vi "apply channel changes.vi"(8 "error in":errorcluster, 9 "new channel":refnum<class "TBM channel.lvclass">, 10 "old channel":refnum<class "TBM channel.lvclass">, 11 "alarms module configuration in":refnum<class "alarms module configuration.lvclass">=refnum) -> (0 "error out":errorcluster, 3 "alarms module configuration out":refnum<class "alarms module configuration.lvclass">)   [LabVIEW 2013]
doc: "Copyright 2016 National Instruments Corporation\n\nLicensed under the Apache License, Version 2.0 (the \"License\"); you may not use this file except in compliance with the License. You may obtain a copy of the License at http://www.apache.org/licenses/LICENSE-2.0\nUnless required by applicable law or agreed to in writing, software distributed under the License is distributed on an \"AS IS\" BASIS, WITHOUT WARRANTIES OR CONDITIONS OF ANY KIND, either express or implied. See the License for the specific language governing permissions and limitations under the License."
uses:
  <vilib>/NI/Tag Bus/tag/tag descriptor.lvclass
  alarms module configuration.lvclass
  <vilib>/NI/Tag Bus Module Framework/channel/TBM channel.lvclass
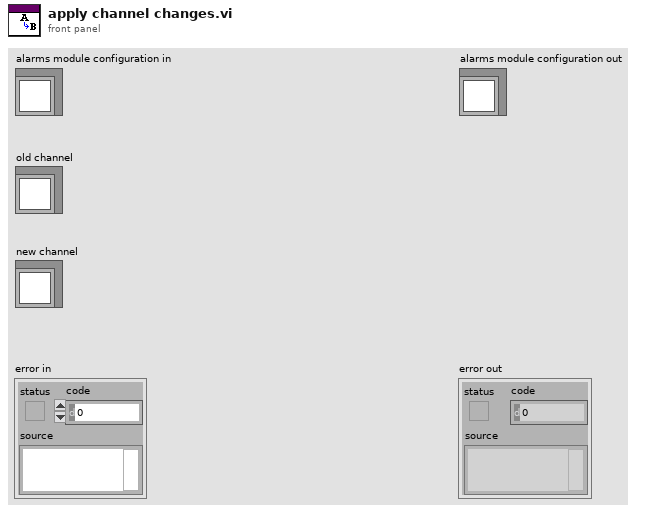
[diagram p1: front panel]
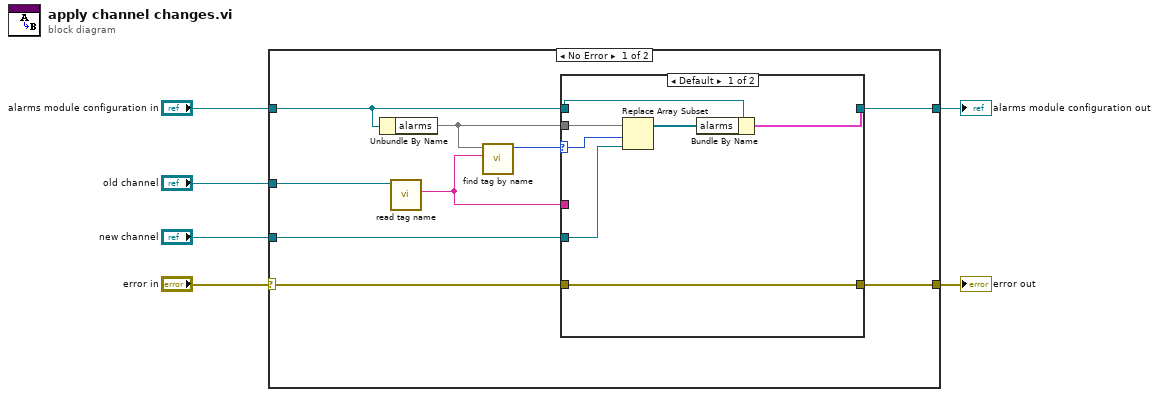
[diagram p0: block diagram]
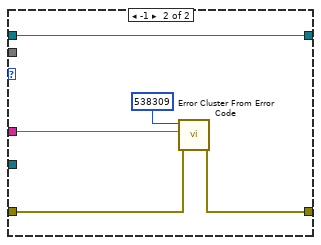
[diagram p2: hidden frame]
diagram:
  n1 = case shown="No Error" "error in" {
    selector: "error in" -> [w10 w29]
    tunnel: [w9 w29] -> w5
    tunnel: [w13 w28] -> w3
    tunnel: "alarms module configuration in" -> [w14 w28]
    tunnel: "old channel" -> [w15 _]
    tunnel: "new channel" -> [w11 _]
    frame No Error {
      n2 = Unbundle By Name(w14) -> ("alarms"=w12)
      n3 = call <vilib>:"read tag name.vi"("system tag in"=w15) -> ("name"=w7:string)  [unwired: 8 in, 2 out]
      n4 = call <vilib>:"find tag by name.vi"("name"=w7, "tags in"=w12) -> ("index"=w8:i32)  [unwired: 9 in]
      n5 = case shown="Default" w8 {
        selector: w8 -> [w20 _]
        tunnel: w14 -> [w22 w27]
        tunnel: [w19 w27] -> w13
        tunnel: w12 -> [w21 _]
        tunnel: w11 -> [w17 _]
        tunnel: w7 -> [_ w25]
        tunnel: w10 -> [w16 w24]
        tunnel: [w16 w23] -> w9
        frame Default {
          n6 = Replace Array Subset(array=w21, new element=w17, index=w20) -> (w18:refnum<class "TBM channel.lvclass">[])
          n7 = Bundle By Name(cluster=w22, "alarms"=w18) -> (w19:cluster{})
        }
        frame -1 {
          n8 = call <vilib>:"Error Cluster From Error Code.vi"("error in (no error)"=w24, "error message (\"\")"=w25, "error code (0)"=538309) -> ("error out"=w23:errorcluster)  [unwired: 6 in]
        }
      }
    }
    frame Error {
    }
  }
  "error out" <- w5
  "alarms module configuration out" <- w3
